vi "rms_analog_input_multichannel_consumer.vi"(4 "Sampling Window [s]":dbl, 6 "Sampling Frequency [Hz]":dbl=2500.0, 7 "Number of Channels":i32, 8 "error in (no error)":errorcluster, 11 "queue out":refnum<queue>) -> (0 "error out":errorcluster, 3 "RMS [V]":dbl[](array[numeric]))   [LabVIEW 2025, in "LabJackEKG.lvlib"]
uses:
  LabJackEKG.lvlib
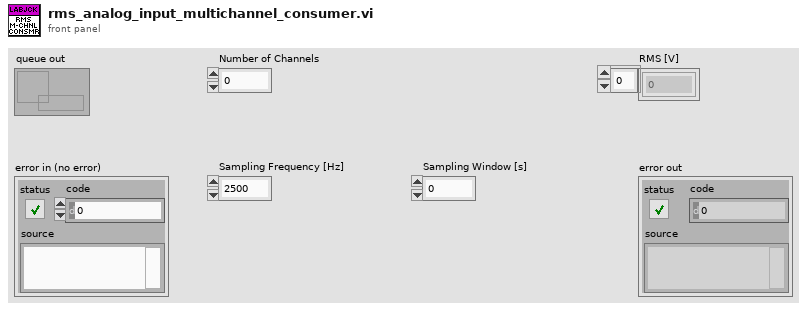
[diagram p1: front panel]
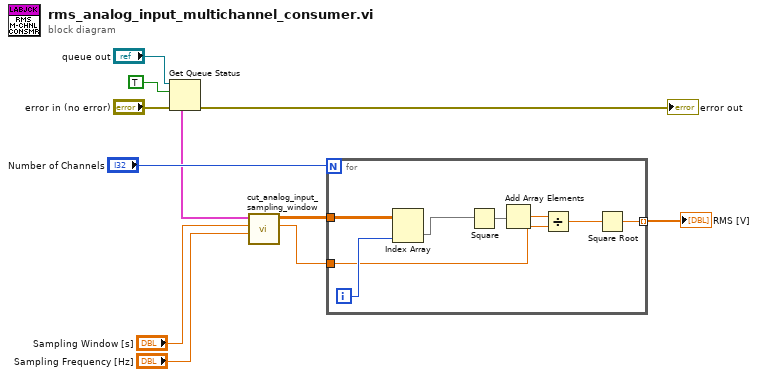
[diagram p0: block diagram]
diagram:
  n1 = Get Queue Status(queue="queue out", return elements? (F)=TRUE, error in (no error)="error in (no error)") -> (error out=→"error out":errorcluster, elements=w1:cluster{"Volt":dbl[]}[])  [unwired: 6 out]
  n2 = call "cut_analog_input_sampling_window.vi"("Sampling Frequency [Hz]"="Sampling Frequency [Hz]", "Sampling Window [s]"="Sampling Window [s]", "elements"=w1) -> ("Window Size"=w7:dbl, "Volt"=w5:dbl[][])  [unwired: 7 in]
  n3 = for {
    N: "Number of Channels" -> [_]
    tunnel: [w17] -> w6 mode=indexing
    tunnel: w5 -> [w15]
    tunnel: w7 -> [w14]
    i -> [w16]
    n4 = Index Array(array=w15, index (col)=w16) -> (element=w13:dbl[])  [unwired: 1 in]
    n5 = Square(x=w13) -> (x^2=w12:dbl[])
    n6 = Add Array Elements(numeric array=w12) -> (sum=w18:dbl)
    n7 = Divide(x=w18, y=w14) -> (x/y=w19:dbl)
    n8 = Square Root(x=w19) -> (sqrt(x)=w17:dbl)
  }
  "RMS [V]" <- w6
